vi "init_pass_buoys.vi"(9 "Buoy Pass 2":T1 {"North" format="%#_10f"; "East" format="%#_8f"}, 11 "Buoy Pass 1":T1 {"North" format="%#_10f"; "East" format="%#_8f"}) -> (2 "Mission.lvclass":refnum<class "Mission.lvclass">)   [LabVIEW 2011, in "Mission.lvclass"]
uses:
  Mission.lvclass
  2 Typedefs/UTM Location.ctl
  Mission.lvclass/Mission.ctl
panel:
  in  "Mission In":refnum<class "Mission.lvclass">
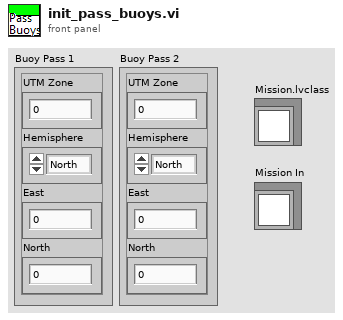
[diagram p1: front panel]
types:
  T1 = typedef "UTM Location.ctl" = cluster{"UTM Zone":dbl, "Hemisphere":enum16{"North", "South"}, "East":dbl, "North":dbl}
  T2 = enum16{"Round Buoy", "Drive", "Pass Buoys", "Station Keeping"}
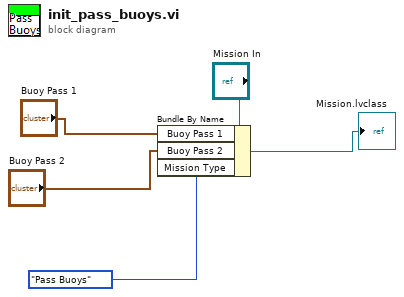
[diagram p0: block diagram]
diagram:
  n1 = Bundle By Name(cluster="Mission In", "Buoy Pass 1"="Buoy Pass 1", "Buoy Pass 2"="Buoy Pass 2", "Mission Type"=T2."Pass Buoys") -> (→"Mission.lvclass":refnum<class "Mission.lvclass">)
